vi "Read.vi"(8 "error in (no error)":errorcluster, 9 "Hit rate warning":refnum<vi>, 10 "Queue overflow indicator":refnum<vi>, 11 "TDCManager refnum":T1) -> (0 "error out":errorcluster)   [LabVIEW 2016]
uses:
  HPTDC Driver Library Folder/Library files/Typedefs/TDCManagerRefnum.ctl
  HPTDC Driver Library Folder/Library files/Typedefs/TDCManager.ctl
  C:/Users/CRT Controller/CRTC Labview Application/Source/HPTDC Driver Library Folder/Library files/hptdc_net4_3.7.0_x64.dll
  HPTDC Driver Library Folder/Library files/hptdc_net4_3.7.0_x64.dll
  HPTDC Driver Library Folder/Library files/Typedefs/TDCHit.ctl
  Global Variables/System info.vi
  Global Variables/Program load indicators.vi
  HPTDC Driver Library Folder/HPTDC Driver Library.lvlib
panel:
  out "Hit rate too great?":bool
  out "timed out?":bool
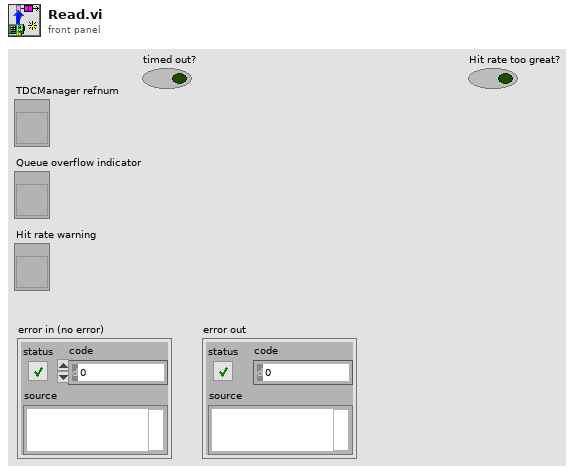
[diagram p1: front panel]
types:
  T1 = typedef "TDCManagerRefnum.ctl" = refnum<vi>
  T2 = typedef "HPTDC Driver Library.lvlib/TDCManager.ctl" = refnum<k24>
  T3 = typedef "HPTDC Driver Library.lvlib/TDCHit.ctl" = cluster{"channel":u8, "time":u64, "type":u8}
  T4 = enum16{"Reset", "ReadAndReset", "Read", "Add", "Init"}
  T5 = typedef "TDCHitArrayPointer.ctl" = refnum<data-value>
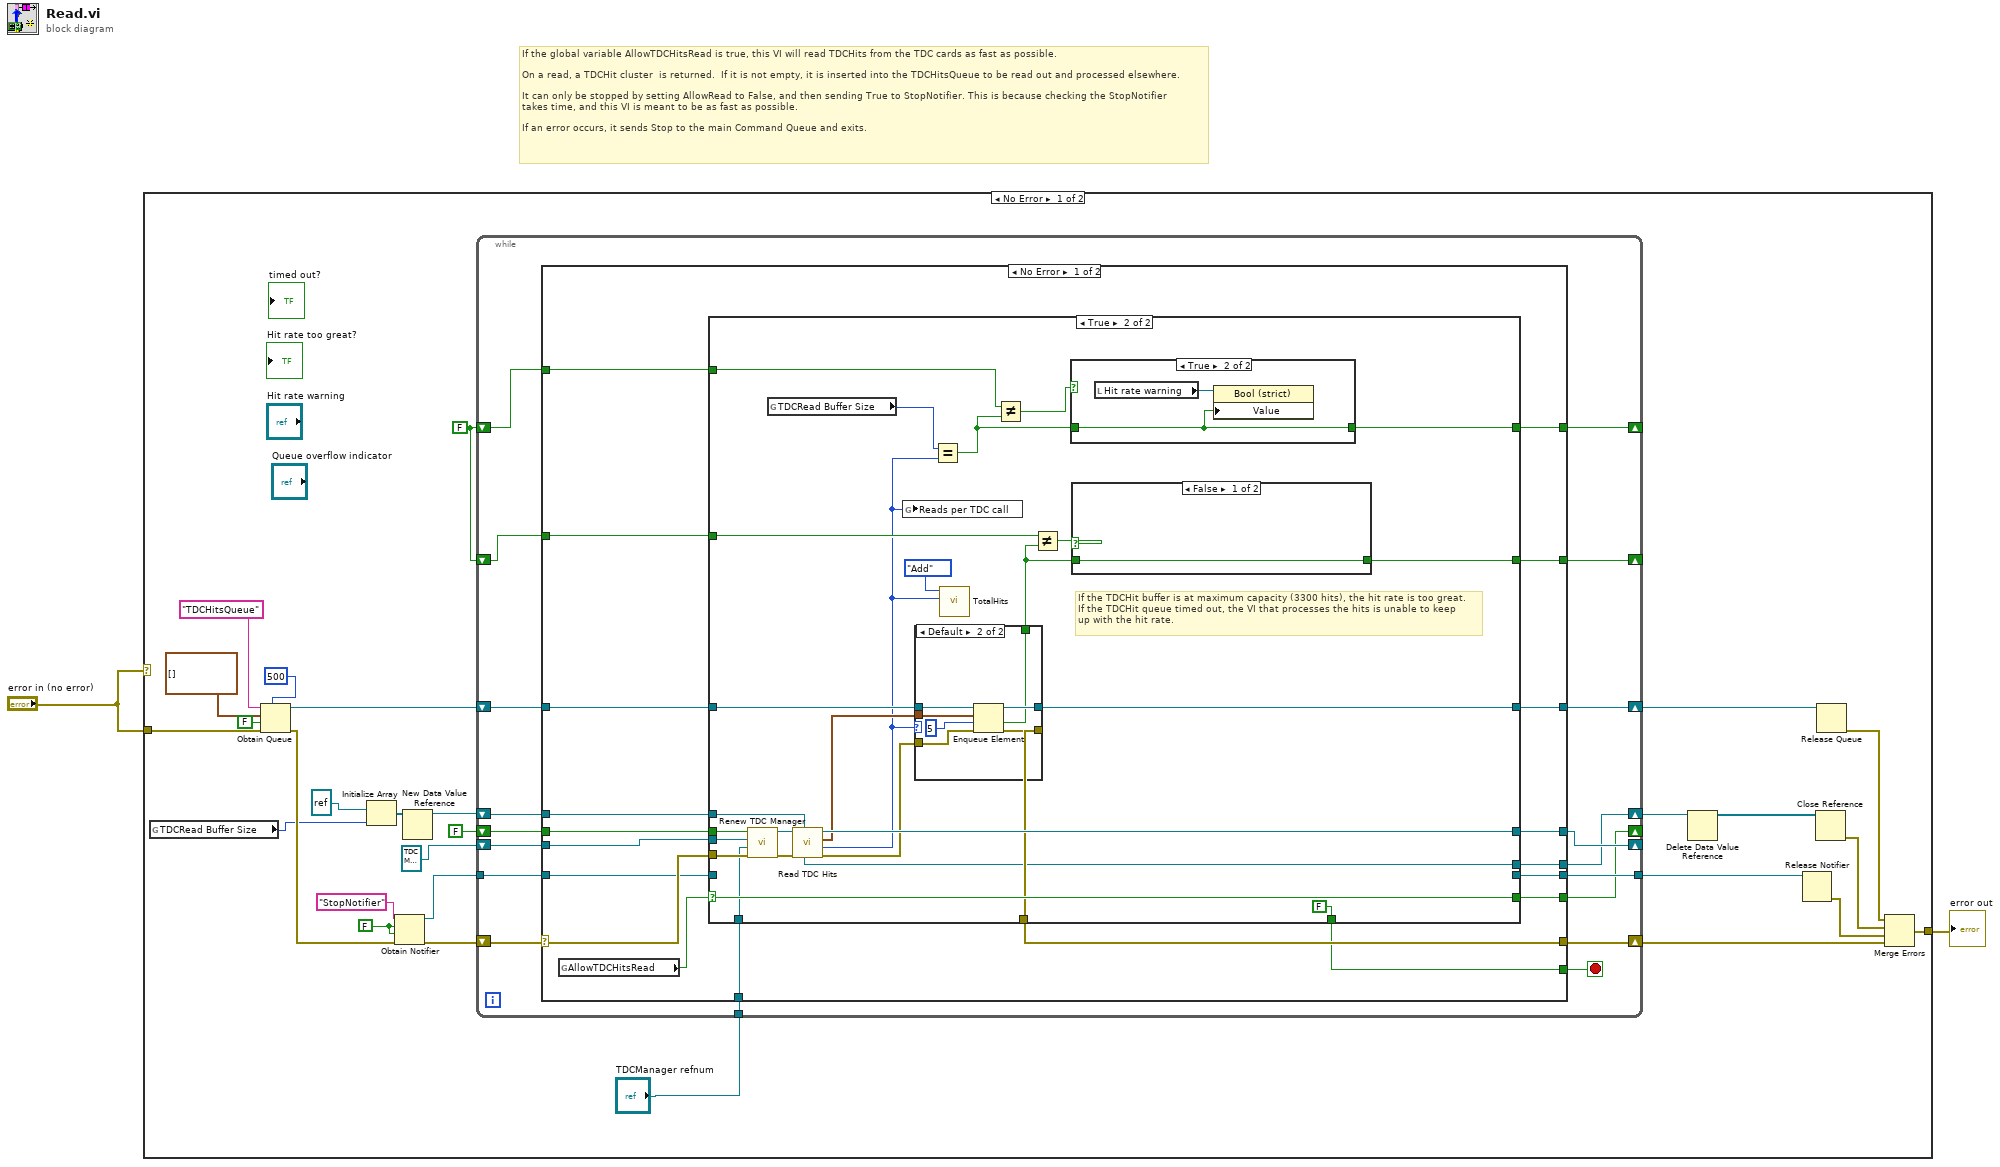
[diagram p0: block diagram]
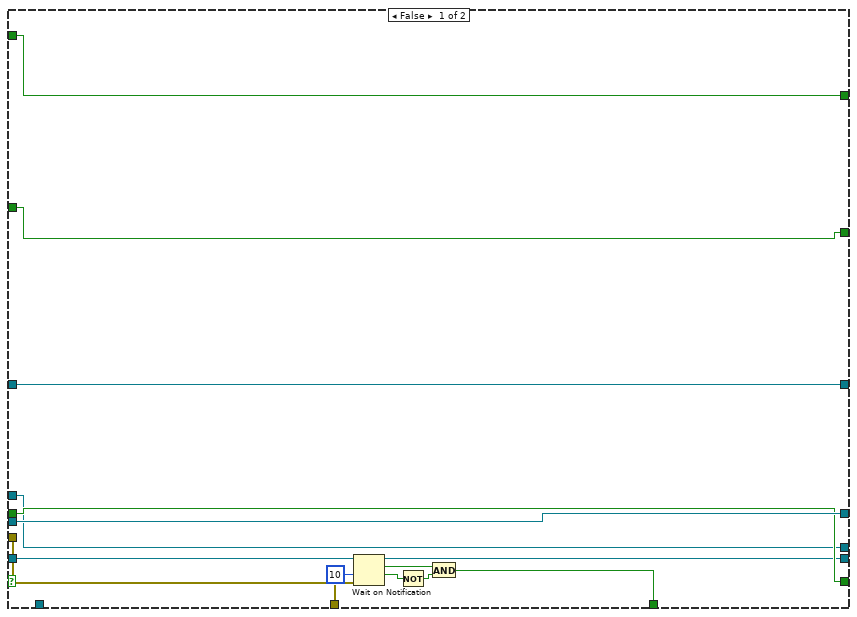
[diagram p2: hidden frame]
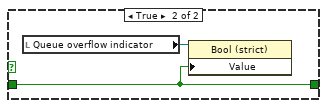
[diagram p3: hidden frame]
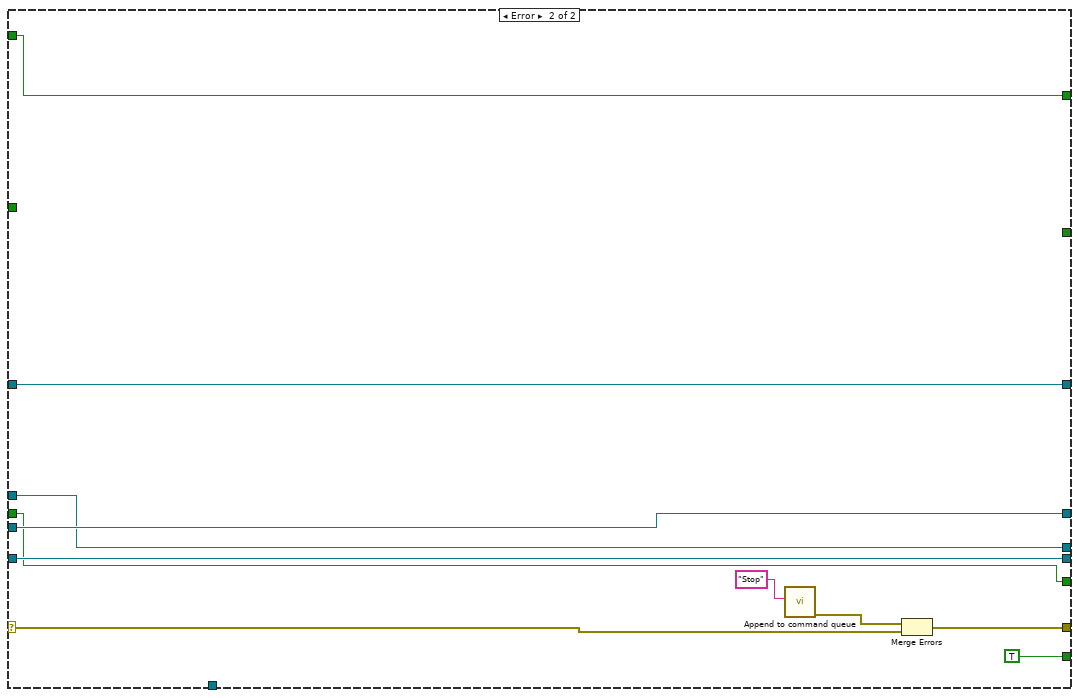
[diagram p6: hidden frame]
diagram:
  # "If the global variable AllowTDCHitsRead is true, this VI will read TDCHits from the TDC cards as fast as possible. \n\nOn a read, a TDCHit cluster  is returned.  If it is not empty, it is inserted into the TDCHitsQueue to be read out and processed elsewhere.\n\nIt can only be stopped by setting AllowRead to False, and then sending True to StopNotifier. This is because checking the StopNotifier\ntakes time, and this VI is meant to be as fast as possible.\n\nIf an error occurs, it sends Stop to the main Command Queue and exits."
  n1 = case shown="No Error" "error in (no error)" {
    tunnel: "error in (no error)" -> [w28 w136]
    tunnel: [w18 w136] -> w2
    frame No Error {
      w10 = FALSE
      w23 = FALSE
      n2 = global read "System info.vi" "TDCRead Buffer Size"() -> (w9:i32)
      n3 = Obtain Queue(max queue size (-1, unlimited)=500, name (unnamed)="TDCHitsQueue", element data type=T3[] [] ("TDCHits"), create if not found? (T)=FALSE, error in (no error)=w28) -> (queue out=w12:refnum<queue>, error out=w14:errorcluster)  [unwired: 1 out]
      n4 = Initialize Array(refnum<k24> refnum (".NET Refnum"), w9) -> (w8:refnum<k24>[])
      n5 = Obtain Notifier(name (unnamed)="StopNotifier", notification data type=w23, create if not found? (T)=w23, error in (no error)=w14) -> (notifier out=w24:refnum<notifier>, error out=w25:errorcluster)  [unwired: 1 out]
      n6 = New Data Value Reference(data value=w8) -> (data value reference=w6:refnum<data-value>)  [unwired: 1 in, 1 out]
      n7 = while {
        shift-right: [w47] -> w15
        shift-left: w25 -> [w42]
        shift-right: [w46] -> _
        shift-left: T2 refnum ("TDCManager") -> [w48]
        shift-right: [w40] -> w21
        shift-left: w12 -> [w41]
        shift-right: [w39] -> _
        shift-left: FALSE -> [w38]
        shift-right: [w36] -> w5
        shift-left: w6 -> [w37]
        tunnel: w24 -> [w45]
        tunnel: [w44] -> w17
        tunnel: "TDCManager refnum" -> [w35]
        shift-right: [w34] -> _
        shift-left: w10 -> [w33]
        shift-right: [w32] -> _
        shift-left: w10 -> [w31]
        stop <- w43 stop-if-true
        n8 = case shown="No Error" w42 {
          selector: w42 -> [w63 w129]
          tunnel: w48 -> [w58 w133]
          tunnel: [w67 w130] -> w47
          tunnel: [w66 w133] -> w46
          tunnel: w45 -> [w53 w134]
          tunnel: [w55 w134] -> w44
          tunnel: [w64 TRUE] -> w43
          tunnel: w41 -> [w62 w128]
          tunnel: [w61 w128] -> w40
          tunnel: [w60 w127] -> w39
          tunnel: w38 -> [w59 w127]
          tunnel: w37 -> [w57 w126]
          tunnel: [w56 w126] -> w36
          tunnel: w35 -> [w54 _]
          tunnel: [w52 w125] -> w34
          tunnel: w33 -> [w51 w125]
          tunnel: [w50 _] -> w32
          tunnel: w31 -> [w49 _]
          frame No Error {
            n9 = global read "AllowTDCHitsRead.vi" "AllowTDCHitsRead"() -> (w65:bool)
            n10 = case shown="True" w65 {
              selector: w65 -> [_ w105]
              tunnel: w58 -> [w82 w100]
              tunnel: w63 -> [w81 w102]
              tunnel: [w80 w98] -> w67
              tunnel: [w82 w109] -> w66
              tunnel: [w75 FALSE] -> w64
              tunnel: w62 -> [w74 w106]
              tunnel: [w74 w103] -> w61
              tunnel: [w73 w105] -> w60
              tunnel: w59 -> [w73 w99]
              tunnel: w57 -> [w72 w84]
              tunnel: [w72 w93] -> w56
              tunnel: [w71 _] -> w55
              tunnel: w54 -> [_ w83]
              tunnel: w53 -> [w70 _]
              tunnel: [w69 w95] -> w52
              tunnel: w51 -> [w69 w94]
              tunnel: [w68 w89] -> w50
              tunnel: w49 -> [w68 w88]
              frame False {
                n11 = Wait on Notification(notifier=w70, timeout in ms (-1)=10, error in (no error)=w81) -> (notifier out=w71:refnum<notifier>, notification=w76:bool, timed out?=w78:bool, error out=w80:errorcluster)  [unwired: 1 in]
                n12 = Not(x=w78) -> (.not. x?=w77:bool)
                n13 = And(x=w76, y=w77) -> (x .and. y?=w75:bool)
              }
              frame True {
                # "If the TDCHit buffer is at maximum capacity (3300 hits), the hit rate is too great.\nIf the TDCHit queue timed out, the VI that processes the hits is unable to keep\nup with the hit rate."
                n14 = call "Renew TDC Manager.vi"("error in"=w102, "TDCManagerRefnum"=w83, "TDCManager"=w100, "Keep old manager?"=w99) -> ("error out"=w101:errorcluster, "TDCManager out"=w104:T2)  [unwired: 6 in]
                n15 = global read "System info.vi" "TDCRead Buffer Size"() -> (w86:i32)
                n16 = call "Read TDC Hits.vi"("data value reference"=w84, "error in (no error)"=w101, "TDCManager"=w104) -> ("error out"=w107:errorcluster, "Hits read"=w85:i32, "Array"=w87:T3[], "TDCManager"=w109:T2, "data value reference out"=w93:T5)  [unwired: 4 in]
                n17 = global write "Program load indicators.vi" "Reads per TDC call"(w85) -> ()
                n18 = case shown="Default" w85 {
                  tunnel: w107 -> [w114 w121]
                  tunnel: w106 -> [w113 w120]
                  tunnel: w87 -> [_ w115]
                  tunnel: [w114 w119] -> w98
                  tunnel: [w113 w117] -> w103
                  tunnel: [_ w116] -> w90
                  frame 0 {
                  }
                  frame Default {
                    n19 = Enqueue Element(queue=w120, element=w115, timeout in ms (-1)=5, error in (no error)=w121) -> (queue out=w117:refnum<queue>, timed out?=w116:bool, error out=w119:errorcluster)
                  }
                }
                n20 = Equal?(x=w86, y=w85) -> (x = y?=w96:bool)
                n21 = call "TotalHits.vi"("Number (0)"=w85, "Action"=T4."Add") -> ()  [unwired: 9 in, 1 out]
                n22 = Not Equal?(x=w94, y=w96) -> (x != y?=w97:bool)
                n23 = Not Equal?(x=w88, y=w90) -> (x != y?=w92:bool)
                n24 = case shown="True" w97 {
                  tunnel: [w122 w124] -> w95
                  tunnel: w96 -> [w122 w124]
                  frame False {
                  }
                  frame True {
                    n25 = local read "Hit rate warning"() -> (w123:refnum<vi>)
                    n26 = property class="Bool (strict)"(reference=w123, "Value"=w124) -> ()  [unwired: 1 in, 2 out]
                  }
                }
                n27 = case shown="False" w92 {
                  tunnel: [w110 w112] -> w89
                  tunnel: w90 -> [w110 w112]
                  frame False {
                  }
                  frame True {
                    n28 = local read "Queue overflow indicator"() -> (w111:refnum<vi>)
                    n29 = property class="Bool (strict)"(reference=w111, "Value"=w112) -> ()  [unwired: 1 in, 2 out]
                  }
                }
              }
            }
          }
          frame Error {
            n30 = call "Append to command queue.vi"("Single command"="Stop") -> ("error out"=w131:errorcluster)  [unwired: 10 in]
            n31 = Merge Errors(w131, w129) -> (w130:errorcluster)
          }
        }
      }
      n32 = Delete Data Value Reference(data value reference=w5) -> (data value=w11:refnum<k24>[])  [unwired: 1 in, 1 out]
      n33 = Release Notifier(notifier=w17) -> (error out=w16:errorcluster)  [unwired: 2 in, 2 out]
      n34 = Close Reference(reference=w11) -> (error out=w20:errorcluster)  [unwired: 1 in]
      n35 = Release Queue(queue=w21) -> (error out=w19:errorcluster)  [unwired: 2 in, 2 out]
      n36 = Merge Errors(w19, w20, w16, w15) -> (w18:errorcluster)
    }
    frame Error {
    }
  }
  "error out" <- w2
